vi "Auto_Routine_StraightTwoPiece.vi"(8 "error in (no error)":errorcluster) -> (0 "error out":errorcluster)   [LabVIEW 2023]
uses:
  Arm2/ArmGetSetpointEnum.ctl
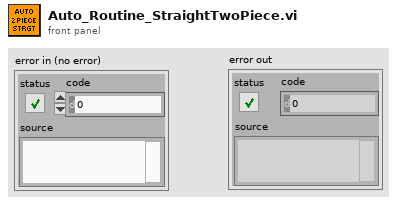
[diagram p1: front panel]
types:
  T1 = typedef "ArmGetSetpointEnum.ctl" = enum16{"ArmFloorPickup", "ArmAmpDeposit", "ArmSpeakerShoot", "ArmStartPosition", "ArmRestPosition", "ArmSourceIntake", "ArmAwayShoot"}
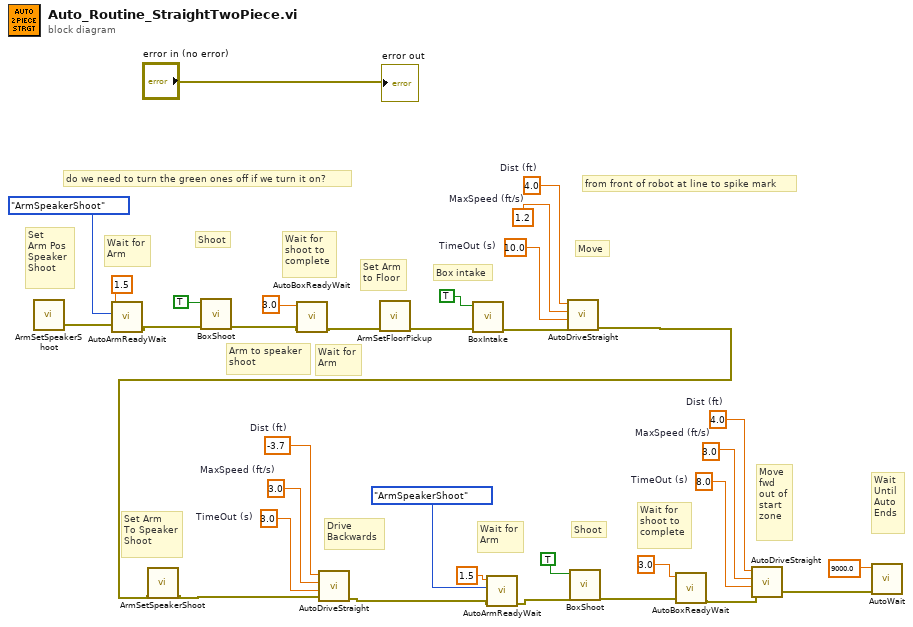
[diagram p0: block diagram]
diagram:
  w31 = 8.0  # TimeOut (s)
  w30 = 3.0  # MaxSpeed (ft/s)
  w29 = 4.0  # Dist (ft)
  w23 = 3.0  # TimeOut (s)
  w22 = 3.0  # MaxSpeed (ft/s)
  w21 = -3.7  # Dist (ft)
  w5 = 10.0  # TimeOut (s)
  w4 = 1.2  # MaxSpeed (ft/s)
  w3 = 4.0  # Dist (ft)
  # "Wait\nUntil\nAuto \nEnds"
  # "Move\nfwd\nout of\nstart\nzone"
  # "Wait for\nshoot to\ncomplete"
  # "Shoot"
  # "Wait for\nArm"
  # "Drive\nBackwards"
  # "Set Arm\nTo Speaker\nShoot"
  # "Wait for\nArm"
  # "Arm to speaker\nshoot"
  # "Box intake"
  # "Move"
  # "Set Arm\nto Floor"
  # "Wait for\nshoot to\ncomplete"
  # "Shoot"
  # "Wait for\nArm"
  # "Set\nArm Pos\nSpeaker\nShoot"
  # "do we need to turn the green ones off if we turn it on?"
  # "from front of robot at line to spike mark"
  n1 = call "ArmSetSpeakerShoot.vi"() -> ("error out"=w11:errorcluster)  [unwired: 11 in]
  n2 = call "AutoArmReadyWait.vi"("error in (no error)"=w11, "ArmSetpoints"=ArmGetSetpointEnum."ArmSpeakerShoot", "TimeOut (s)"=1.5) -> ("error out"=w12:errorcluster)  [unwired: 8 in]
  n3 = call "BoxShoot.vi"("error in (no error)"=w12, "Box shoot"=TRUE) -> ("error out"=w14:errorcluster)  [unwired: 9 in]
  n4 = call "AutoBoxReadyWait.vi"("error in (no error)"=w14, "TimeOut (s)"=3.0) -> ("error out"=w15:errorcluster)  [unwired: 9 in]
  n5 = call "ArmSetFloorPickup.vi"("error in (no error)"=w15) -> ("error out"=w9:errorcluster)  [unwired: 10 in]
  n6 = call "BoxIntake.vi"("error in (no error)"=w9, "Box intake"=TRUE) -> ("error out"=w10:errorcluster)  [unwired: 9 in]
  n7 = call "AutoDriveStraight.vi"("error in (no error)"=w10, "TimeOut (s)"=w5, "MaxSpeed (ft/s)"=w4, "Dist (ft)"=w3) -> ("error out"=w25:errorcluster)  [unwired: 7 in]
  n8 = call "ArmSetSpeakerShoot.vi"("error in (no error)"=w25) -> ("error out"=w26:errorcluster)  [unwired: 10 in]
  n9 = call "AutoDriveStraight.vi"("error in (no error)"=w26, "TimeOut (s)"=w23, "MaxSpeed (ft/s)"=w22, "Dist (ft)"=w21) -> ("error out"=w24:errorcluster)  [unwired: 7 in]
  n10 = call "AutoArmReadyWait.vi"("error in (no error)"=w24, "ArmSetpoints"=ArmGetSetpointEnum."ArmSpeakerShoot", "TimeOut (s)"=1.5) -> ("error out"=w17:errorcluster)  [unwired: 8 in]
  n11 = call "BoxShoot.vi"("error in (no error)"=w17, "Box shoot"=TRUE) -> ("error out"=w27:errorcluster)  [unwired: 9 in]
  n12 = call "AutoBoxReadyWait.vi"("error in (no error)"=w27, "TimeOut (s)"=3.0) -> ("error out"=w32:errorcluster)  [unwired: 9 in]
  n13 = call "AutoDriveStraight.vi"("error in (no error)"=w32, "TimeOut (s)"=w31, "MaxSpeed (ft/s)"=w30, "Dist (ft)"=w29) -> ("error out"=w33:errorcluster)  [unwired: 7 in]
  n14 = call "AutoWait.vi"("error in (no error)"=w33, "TimeOut (s)"=9000.0) -> ()  [unwired: 9 in, 1 out]
  "error out" <- "error in (no error)"
